vi "AlliGator Get Phasor Calibration in Calibration Map.vi"(6 "Calibration Map MD5 Digest":string, 8 "Error In":errorcluster, 9 "Phasor Calibration in":T3, 10 "ROI Center":cluster{"X":i32, "Y":i32}, 11 "Phasor Calibration Map":T1={"Phasor Frequency"=80000000.0, "Calibration Lifetime"=1e-09, "ROI Centers"=[], "ROI Descriptors"=[], "Map Resolution X"=0, "Map Resolution Y"=0, "z Array"=[]} {"ROI Descriptors"."Contours"."Type" items=["No Selection", "Point", "Line", "Rectangle", "Oval", "Polygon", "Freehand Region", "Annulus", "Unused2", "Unused3", "Broken Line", "Freehand Line", "Rotated Rectangle"]}) -> (0 "Error Out":errorcluster, 3 "Phasor Calibration out":T3)   [LabVIEW 2021, in "AlliGator Phasor Calibration.lvlib"]
doc: "Finds the <B>Phasor Calibration</B> corresponding to the <B>ROI Center</B> location.\n\nIf the location corresponds to a \"dummy\" ROI (typically a phasor created by manual conversion of a decay into a phasor by user interaction), the <B>Phasor Calibration in</B> is used."
uses:
  AlliGator Phasor Calibration.lvlib
  AlliGator Settings.lvlib
  AlliGator Settings List.ctl
  Variant/Variant to Data/Variant to Data.lvlib
  Utilities/Utilities.lvlib
  6d308cf6-a12b-4f13-a66f-4b3b86bda0cd.vi
  Phasor/Calibration Phasor (m, phi).ctl
  Phasor/Phasor.lvlib
  Phasor/Phasor Calibration Map v2.ctl
panel:
  # "see the AlliGator License on the block diagram (Ctrl+E or Window:Show Block Diagram)"
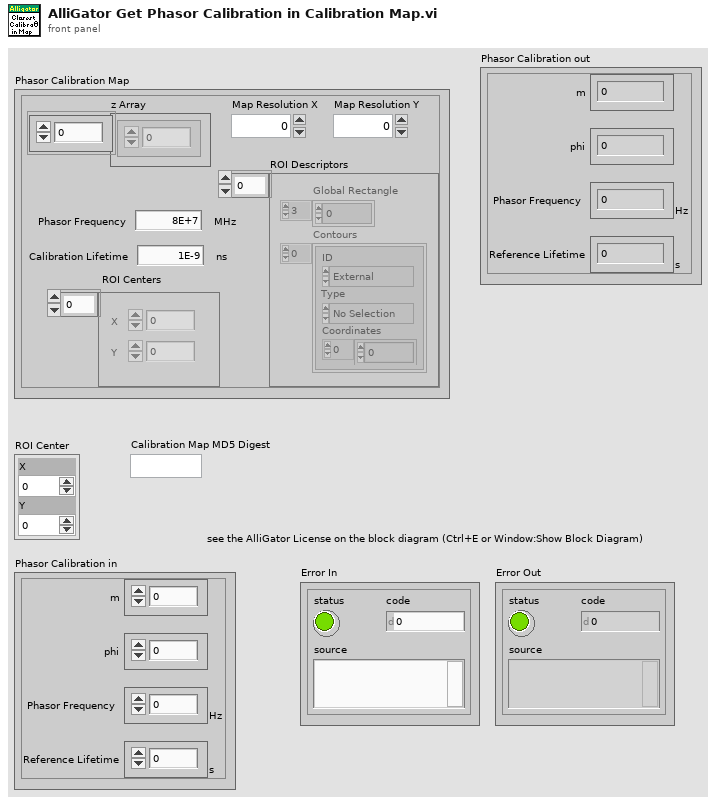
[diagram p1: front panel]
types:
  T1 = typedef "Phasor.lvlib/Phasor Calibration Map v2.ctl" = cluster{"Phasor Frequency":dbl[unit], "Calibration Lifetime":dbl[unit], "ROI Centers":cluster{"X":i32, "Y":i32}[], "ROI Descriptors":T2[], "Map Resolution X":i32, "Map Resolution Y":i32, "z Array":cdb[]}
  T2 = typedef "ROI Descriptor" = cluster{"Global Rectangle":i32[], "Contours":cluster{"ID":enum32{"External", "Internal"}, "Type":u32, "Coordinates":i32[]}[]}
  T3 = typedef "Phasor.lvlib/Calibration Phasor (m, phi).ctl" = cluster{"m":dbl, "phi":dbl, "Phasor Frequency":dbl[unit], "Reference Lifetime":dbl[unit]}
  T4 = typedef "AlliGator Settings.lvlib/AlliGator Settings List.ctl" = enum16{"GUI:Visible Settings Tab", "GUI:Last Run Version", "Source Image:Use Image Histogram for Contrast", "Source Image:Low Count Pixels Rejection Options", "Source Image:High Count Pixels Rejection Options", "Source Image:Use Image Brightness", "Source Image:Blend Overlay with Image Background", "Source Image:Use Fixed ROI Diameter", "Source Image:ROI Diameter", "Source Image:ROI Center Color", "Source Image:Peak Threshold", "Source Image:Intensity Threshold", "Source Image:Image Binning Options", "Source Image:Image Smoothing Options", "Source Image:Image Histogram Active", "Source Image:Invert Binary Mask", "Source Image:Hot Pixel Removal", "Source Image:Overlay Analyzed ROI Center", "Source Image:Auto-Adjust Contrast", "Source Image:Histogram Lower Percentile", "Source Image:Histogram Upper Percentile", "Source Image:Save Source Image", "Source Image:Scale Bar Options", "Source Image:Image Resolution (Pixel Size)", "Source Image:Flatfield Correction", "Data Information:Gate Width", "Data Information:Nanotime Gate Separation", "Data Information:Macrotime Gate Separation", "Data Information:Gate Step", "Data Information:# Gates", "Data Information:Gate Image Exposure", "Data Information:Gate Image Integration", "Data Information:Gates to Skip", "Data Information:Gates to Keep", "Data Information:Define Gates to", "Data Information:Channel Name", "Data Information:Available Channel Names", "Data Information:Channel Arithmetic", "Data Information:Background File Subtraction", "Data Information:Background File", "Data Information:Background Scaling Factor", "Data Information:Background Pile-up Correction", "Data Information:Background Pixel Well Capacity", "Data Information:Laser Period", "Data Information:SYNC Period", "Data Information:Pile-up Correction", "Data Information:Pixel Well Capacity", "Data Information:Dataset Scaling Factor", "Fluorescence Decay_Decay Pre-Processing:Reverse Gates", "Fluorescence Decay_Decay Pre-Processing:Verbose Decay Pre-Processing", "Fluorescence Decay_Decay Pre-Processing:Use Decay Pre-Processing", "Fluorescence Decay_Decay Pre-Processing:Background Subtraction", "Fluorescence Decay_Decay Pre-Processing:Background Definition Range", "Fluorescence Decay_Decay Pre-Processing:Baseline Subtraction Method", "Fluorescence Decay_Decay Pre-Processing:Operations Order", "Fluorescence Decay_Decay Pre-Processing:Smoothing Parameter", "Fluorescence Decay_Decay Pre-Processing:Shift Decay", "Fluorescence Decay_Decay Pre-Processing:Decay Shift Parameters", "Fluorescence Decay_Decay Pre-Processing:Fold Decay", "Fluorescence Decay_Decay Pre-Processing:# Folds", "Fluorescence Decay_Decay Pre-Processing:1-Normalize Decay", "Fluorescence Decay_Decay Pre-Processing:[0-1]-Normalize Decay", "Fluorescence Decay_Decay Pre-Processing:Smoothen Decay", "Fluorescence Decay_Decay Pre-Processing:Extrapolate Decay", "Fluorescence Decay_Decay Pre-Processing:Use Periodicity", "Fluorescence Decay_Decay Pre-Processing:Use Cursors", "Fluorescence Decay_Decay Pre-Processing:Tail Fraction", "Fluorescence Decay_Decay Pre-Processing:Head Fraction", "Fluorescence Decay_Decay Pre-Processing:Additional Points", "Fluorescence Decay_Decay Pre-Processing:Straighten Decay", "Fluorescence Decay_Decay Pre-Processing:Constant Background", "Fluorescence Decay_Decay Pre-Processing:Pixel-Normalize Decay", "Fluorescence Decay_Advanced Analysis:Extract IRF instead of Decay", "Fluorescence Decay_Advanced Analysis:IRF Extraction Options", "Fluorescence Decay_Advanced Analysis:IRF Optimization Options", "Fluorescence Decay_Advanced Analysis:Square Pulse Options", "Fluorescence Decay_Advanced Analysis:IRF Order", "Fluorescence Decay_Advanced Analysis:IRF Time Constants", "Fluorescence Decay_Advanced Analysis:Wavelet Analysis Options", "Fluorescence Decay_Advanced Analysis:Average Lifetime Options", "Fluorescence Decay_Fit Options:Fit Options", "Fluorescence Decay_Fit Options:Use Legacy Fitting Approach", "Fluorescence Decay_Fit Options:Use Data Information Laser Period", "Fluorescence Decay_Fit Parameters:Displayed Fit Parameters", "Fluorescence Decay_Fit Parameters:Fit Parameter Constraints", "Fluorescence Decay_Fit Parameters:Export Tabulated Results", "Fluorescence Decay_Fit Parameters:MLE Baseline Offset Type", "Fluorescence Decay_Fit Parameters:MLE Baseline Offset", "Fluorescence Decay_Fit Parameters:Guess Parameter Names", "Fluorescence Decay_Fit Parameters:Guess Parameter Values", "Fluorescence Decay_Fit Parameters:Guess Parameters Options", "Fluorescence Decay_Styles:Show Last Decay Only", "Fluorescence Decay_Styles:Decay Graph Color Array", "Fluorescence Decay:Decay Graph Active", "Fluorescence Decay Statistics:Min Peak Value", "Fluorescence Decay Statistics:Reject Low Decay Peak Pixels", "Fluorescence Decay Statistics:Reject High Decay Peak Pixels", "Fluorescence Decay Statistics:Max Peak Value", "Time Traces:Use File Timestamp", "Time Traces:Time Step", "Time Traces:Use Intensity Correction File", "Time Traces:Intensity Correction File", "Phasor Plot:Phasor Plot Smoothing Options", "Phasor Plot:Phasor Plot Size", "Phasor Plot:Phasor Plot Graphics Options", "Phasor Plot:Cumulative Phasor Plot", "Phasor Plot:Use Phasor Brightness", "Phasor Plot:Blend Overlay with Phasor Background", "Phasor Plot:Save Phasor Plot", "Phasor Plot:Show References", "Phasor Plot:Phasor Ratio Decay Range", "Phasor Plot:Exponential Fading", "Phasor Plot:Phasor Ratio Reference Colors", "Phasor Plot:Reference Radius", "Phasor Plot:Show Color Map Vertices", "Phasor Plot:Phasor Plot Active", "Phasor Plot:Phasor Ratio Color Map Type", "Phasor Plot:Phasor Ratio Color Map", "Phasor Plot:Phasor Ratio Display Range", "Phasor Plot:Selected Image ROI(s)", "Phasor Plot:All Image ROIs", "Phasor Plot:Selected Phasor Plot ROI(s)", "Phasor Plot:All Phasor Plot ROIs", "Phasor Plot:Phasor Ratio Color-Coded Quantity", "Phasor Plot:Store Phasor Harmonics", "Phasor Plot:Draw Reference Segment", "Phasor Plot:User-Defined Quantity", "Phasor Graph:Phasor Frequency", "Phasor Graph:Phasor Ratio Type", "Phasor Graph:Pixel-level Phasor Computation", "Phasor Graph:Save Phasor Graph", "Phasor Graph:Phasor Graph Active", "Phasor Graph:Phasor SDV Options", "Phasor Calibration:Use Backup Calibration if needed", "Phasor Graph:Define Shortest Lifetime as", "Phasor Calibration:Backup Calibration Type", "Phasor Calibration:Calibration Type", "Phasor Calibration:Calibration Lifetime", "Phasor Calibration:Calibration Map Algorithm", "Single-Exponential Phasor Locus (SEPL):Gate Parameters", "Single-Exponential Phasor Locus (SEPL):User-defined Gate", "Single-Exponential Phasor Locus (SEPL):User-defined IRF", "Single-Exponential Phasor Locus (SEPL):Phasor Parameters", "Single-Exponential Phasor Locus (SEPL):Decay & IRF Parameters", "Single-Exponential Phasor Locus (SEPL):Display Parameters", "Lifetime Analysis:Decay Analysis Parameters", "Lifetime Analysis:Lifetime Map Active", "Plugins:Python Settings", "Miscellaneous:Verbose Mode", "Miscellaneous:Beep after Script", "Miscellaneous:Saved Image File Format", "Miscellaneous:Exported Gate Image Settings", "Miscellaneous:Include Loading in Timing", "Miscellaneous:Verbose Settings Mode", "Miscellaneous:Histogram Options", "Miscellaneous:Beep on Error", "Miscellaneous:# Logical Processors Used", "Miscellaneous:ROI Description Max Characters", "Miscellaneous:Verbose Error Mode", "Miscellaneous:Transparent Mask Color"}
  T5 = enum16{"Single Calibration", "Nearest Valid Calibration"}
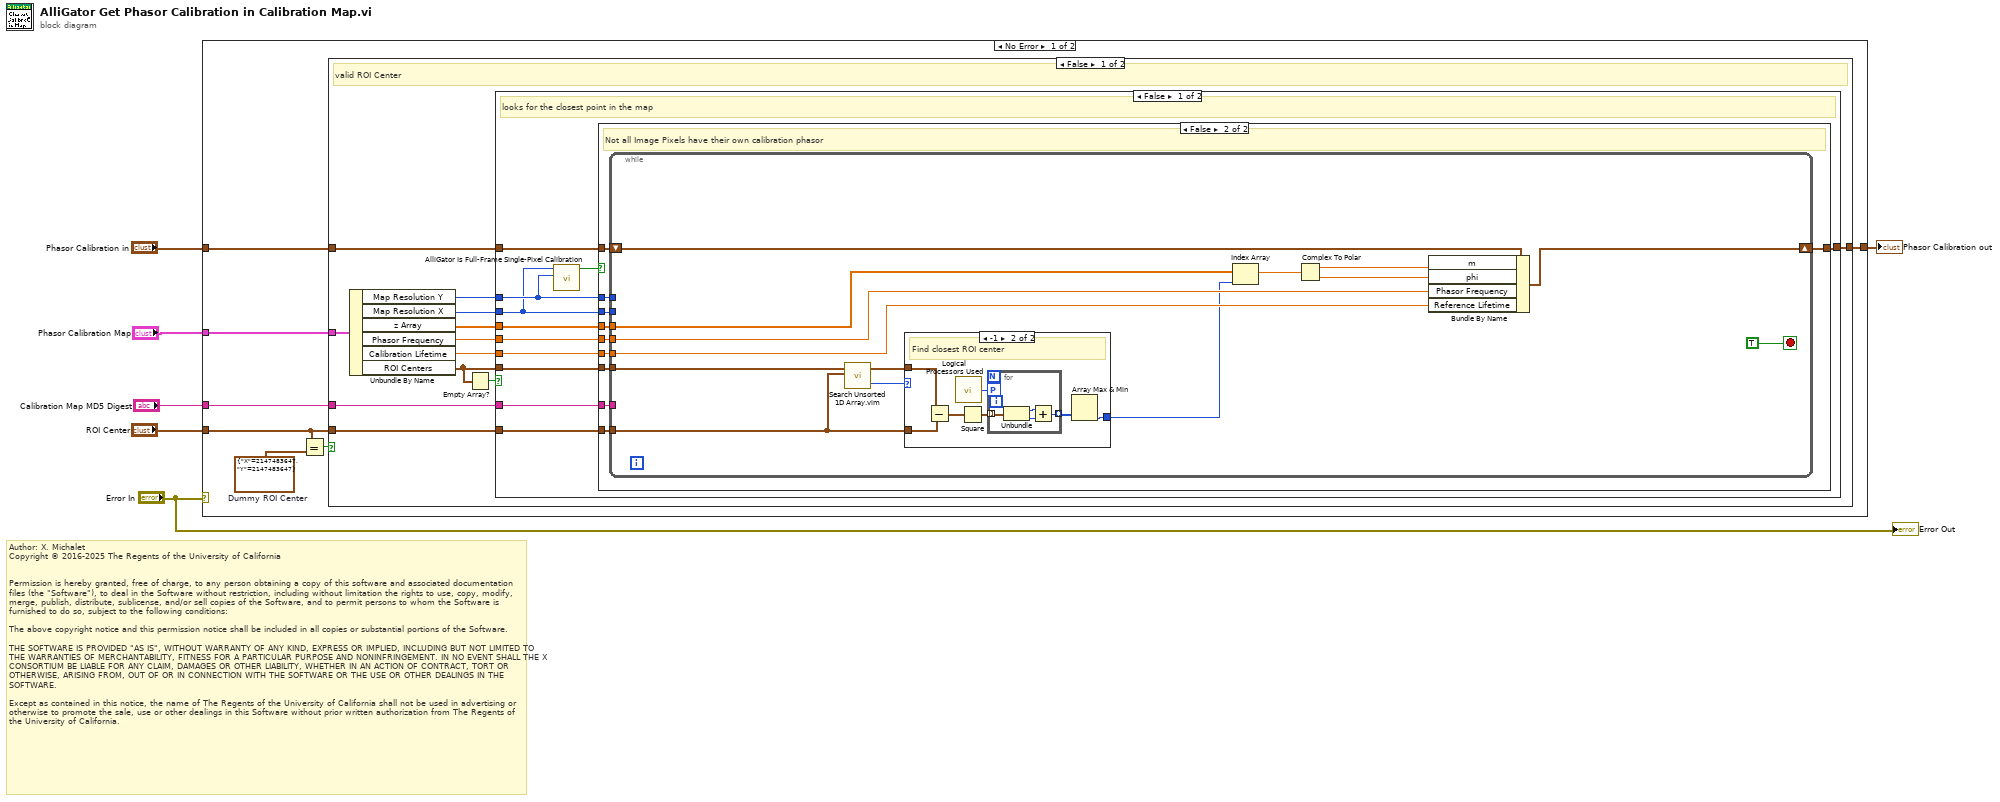
[diagram p0: block diagram]
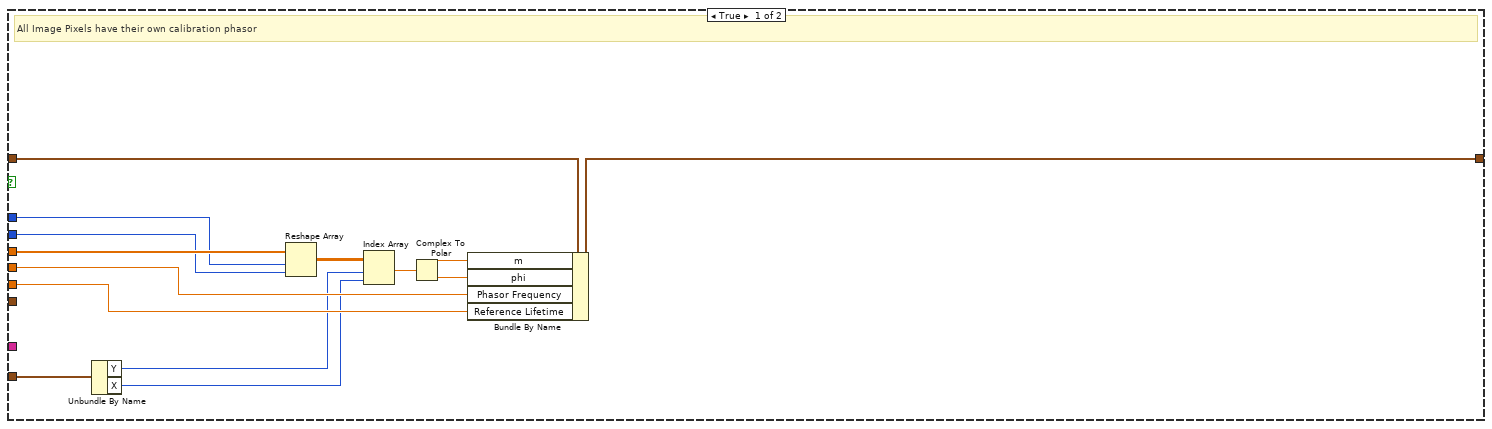
[diagram p2: hidden frame]
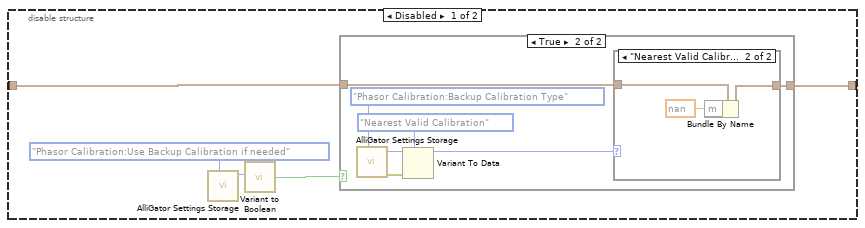
[diagram p6: hidden frame]
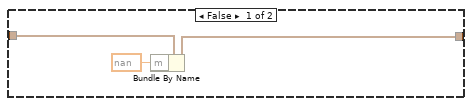
[diagram p7: hidden frame]
diagram:
  # "Author: X. Michalet\nCopyright © 2016-2025 The Regents of the University of California\n \n\nPermission is hereby granted, free of charge, to any person obtaining a copy of this software and associated documentation files (the \"Software\"), to deal in the Software without restriction, including without limitation the rights to use, copy, modify, merge, publish, distribute, sublicense, and/or sell copies of the Software, and to permit persons to whom the Software is furnished to do so, subject to the following conditions:\n\nThe above copyright notice and this permission notice shall be included in all copies or substantial portions of the Software.\n\nTHE SOFTWARE IS PROVIDED \"AS IS\", WITHOUT WARRANTY OF ANY KIND, EXPRESS OR IMPLIED, INCLUDING BUT NOT LIMITED TO THE WARRANTIES OF MERCHANTABILITY, FITNESS FOR A PARTICULAR PURPOSE AND NONINFRINGEMENT. IN NO EVENT SHALL THE X CONSORTIUM BE LIABLE FOR ANY CLAIM, DAMAGES OR OTHER LIABILITY, WHETHER IN AN ACTION OF CONTRACT, TORT OR OTHERWISE, ARISING FROM, OUT OF OR IN CONNECTION WITH THE SOFTWARE OR THE USE OR OTHER DEALINGS IN THE SOFTWARE.\n\nExcept as contained in this notice, the name of The Regents of the University of California shall not be used in advertising or otherwise to promote the sale, use or other dealings in this Software without prior written authorization from The Regents of the University of California."
  n1 = case shown="No Error" "Error In" {
    tunnel: "Phasor Calibration Map" -> [w13 _]
    tunnel: "ROI Center" -> [w9 _]
    tunnel: "Phasor Calibration in" -> [w12 w109]
    tunnel: [w11 w109] -> w3
    tunnel: "Calibration Map MD5 Digest" -> [w7 _]
    frame No Error {
      w10 = cluster{"X":i32, "Y":i32} {"X"=2147483647, "Y"=2147483647}  # Dummy ROI Center
      n2 = Equal?(x=w9, y=w10) -> (x = y?=w8:bool)
      n3 = case shown="False" w8 {
        tunnel: w13 -> [w19 _]
        tunnel: w12 -> [w24 w88]
        tunnel: [w23 w87] -> w11
        tunnel: w9 -> [w20 _]
        tunnel: w7 -> [w17 _]
        frame False {
          # "valid ROI Center"
          n4 = Unbundle By Name(w19) -> ("Map Resolution Y"=w15:i32, "Map Resolution X"=w14:i32, "z Array"=w16:cdb[], "Phasor Frequency"=w22:dbl[unit], "Calibration Lifetime"=w21:dbl[unit], "ROI Centers"=w18:cluster{"X":i32, "Y":i32}[])
          n5 = Empty Array?(array=w18) -> (empty?=w25:bool)
          n6 = case shown="False" w25 {
            tunnel: w24 -> [w36 w86]
            tunnel: [w35 w86] -> w23
            tunnel: w22 -> [w34 _]
            tunnel: w21 -> [w33 _]
            tunnel: w20 -> [w32 _]
            tunnel: w18 -> [w29 _]
            tunnel: w17 -> [w31 _]
            tunnel: w16 -> [w30 _]
            tunnel: w15 -> [w28 _]
            tunnel: w14 -> [w27 _]
            frame False {
              # "looks for the closest point in the map"
              n7 = call "AlliGator Is Full-Frame Single-Pixel Calibration.vi"("Map Resolution Y"=w28, "Map Resolution X"=w27) -> ("Full-Frame Single-Pixel Calibration?"=w26:bool)  [unwired: 8 in, 1 out]
              n8 = case shown="False" w26 {
                tunnel: w36 -> [w50 w60]
                tunnel: [w49 w59] -> w35
                tunnel: w34 -> [w48 w58]
                tunnel: w33 -> [w47 w57]
                tunnel: w32 -> [w46 w56]
                tunnel: w29 -> [_ w55]
                tunnel: w31 -> [_ w54]
                tunnel: w30 -> [w45 w53]
                tunnel: w28 -> [w44 w52]
                tunnel: w27 -> [w43 w51]
                frame True {
                  # "All Image Pixels have their own calibration phasor"
                  n9 = Unbundle By Name(w46) -> ("Y"=w41:i32, "X"=w40:i32)
                  n10 = Reshape Array(w45, w44, w43) -> (w42:cdb[][])
                  n11 = Index Array(array=w42, index (row)=w41, index (col)=w40) -> (element=w39:cdb)
                  n12 = Complex To Polar(r * e^(i*theta)=w39) -> (r=w38:dbl, theta=w37:dbl)
                  n13 = Bundle By Name(cluster=w50, "m"=w38, "phi"=w37, "Phasor Frequency"=w48, "Reference Lifetime"=w47) -> (w49:T3)
                }
                frame False {
                  # "Not all Image Pixels have their own calibration phasor"
                  n14 = while {
                    tunnel: w58 -> [w71]
                    tunnel: w57 -> [w70]
                    tunnel: w56 -> [w69]
                    tunnel: w55 -> [w68]
                    tunnel: w54 -> [_]
                    tunnel: w53 -> [w67]
                    tunnel: w52 -> [_]
                    tunnel: w51 -> [_]
                    shift-right: [w72] -> w59
                    shift-left: w60 -> [w73]
                    stop <- TRUE stop-if-true
                    n15 = call "Search Unsorted 1D Array.vim"("element"=w69, "unsorted 1D array"=w68) -> ("index of element"=w61:i32)  [unwired: 9 in]
                    n16 = case shown="-1" w61 {
                      selector: w61 -> [w74 _]
                      tunnel: [w74 w81] -> w64
                      tunnel: w68 -> [_ w78]
                      tunnel: w69 -> [_ w77]
                      frame 0, Default {
                        # "If found, use it"
                      }
                      frame -1 {
                        # "Find closest ROI center"
                        n17 = Subtract(x=w78, y=w77) -> (x-y=w75:cluster{"X":i32, "Y":i32}[])
                        n18 = call "Logical Processors Used.vi"() -> ("# Logical Processor Used"=w76:i32)  [unwired: 6 in]
                        n19 = Square(x=w75) -> (x^2=w80:cluster{"X":i32, "Y":i32}[])
                        n20 = for {
                          tunnel: w80 -> [w85] mode=indexing
                          tunnel: [w82] -> w79 mode=indexing
                          workers-P: w76 -> [_]
                          n21 = Unbundle(w85) -> ("X"=w84:i32, "Y"=w83:i32)
                          n22 = Add(x=w84, y=w83) -> (x+y=w82:i32)
                        }
                        n23 = Array Max & Min(array=w79) -> (min index (indices)=w81:i32)  [unwired: 3 out]
                      }
                    }
                    n24 = Index Array(array=w67, index=w64) -> (element=w65:cdb)
                    n25 = Complex To Polar(r * e^(i*theta)=w65) -> (r=w63:dbl, theta=w62:dbl)
                    n26 = Bundle By Name(cluster=w73, "m"=w63, "phi"=w62, "Phasor Frequency"=w71, "Reference Lifetime"=w70) -> (w72:T3)
                  }
                }
              }
            }
            frame True {
              # "empty calibration map: used stored calibration"
            }
          }
        }
        frame True {
          # "if ROI Center is NaN (e.g. user-entered decay to phasor conversion) use default calibration"
          n27 = disable-structure shown="Enabled" {
            disable-tunnel: w88 -> [w90 w108]
            disable-tunnel: [w89 w108] -> w87
            frame Disabled {
              n28 = call "AlliGator Settings Storage.vi"("AlliGator Settings List"=AlliGator_Settings_List."Phasor Calibration:Use Backup Calibration if needed") -> ("Variant Data out"=w93:variant)  [unwired: 9 in, 1 out]
              n29 = call "Variant to Boolean.vi"("Variant"=w93) -> ("Value"=w91:bool)  [unwired: 8 in]
              n30 = case shown="True" w91 {
                tunnel: w90 -> [w96 w98]
                tunnel: [w95 w97] -> w89
                frame False {
                  n31 = Bundle By Name(cluster=w96, "m"=nan) -> (w95:T3)
                }
                frame True {
                  n32 = call "AlliGator Settings Storage.vi"("AlliGator Settings List"=AlliGator_Settings_List."Phasor Calibration:Backup Calibration Type") -> ("Error Out"=w102:errorcluster, "Variant Data out"=w101:variant)  [unwired: 9 in]
                  n33 = Variant To Data(error in=w102, type=T5."Nearest Valid Calibration" ("Backup Calibration"), Variant=w101) -> (data=w99:T5)  [unwired: 1 out]
                  n34 = case shown="\"Nearest Valid Calibration\"" w99 {
                    tunnel: w98 -> [w104 w107]
                    tunnel: [w104 w106] -> w97
                    frame "Single Calibration", Default {
                    }
                    frame "Nearest Valid Calibration" {
                      n35 = Bundle By Name(cluster=w107, "m"=nan) -> (w106:T3)
                    }
                  }
                }
              }
            }
            frame Enabled {
            }
          }
        }
      }
    }
    frame Error {
    }
  }
  "Phasor Calibration out" <- w3
  "Error Out" <- "Error In"
